vi "test Get Device ID.vi"(11 "Test Case In":refnum<class "Test PCANBasic.lvclass">) -> (0 "error out":errorcluster, 3 "Test Case Out":refnum<class "Test PCANBasic.lvclass">)   [LabVIEW 2020, in "Test PCANBasic.lvclass"]
uses:
  Test PCANBasic.lvclass
  C:/Program Files/National Instruments/LabVIEW 2025/vi.lib/Astemes/LUnit/Test Case.lvclass
  <vilib>/Astemes/LUnit/Test Case.lvclass/Test Case.ctl
  source/PCANBasic.lvlib
  Global PCAN Channel.vi
  <vilib>/Astemes/LUnit/Test Case.lvclass
panel:
  out "Device ID":u32
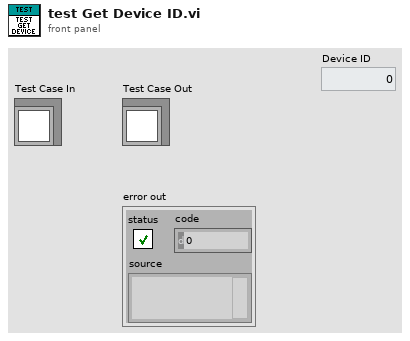
[diagram p1: front panel]
types:
  T1 = typedef "PCANBasic.lvlib/TPCANHandle.ctl" = u16
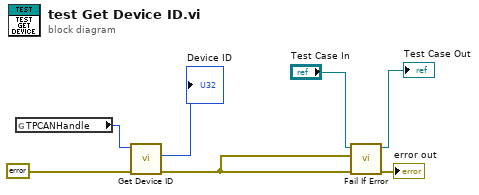
[diagram p0: block diagram]
diagram:
  n1 = global read "Global PCAN Channel.vi" "TPCANHandle"() -> (w2:T1)
  n2 = call "Get Device ID.vi"("error in"=errorcluster {"status"=FALSE, "code"=0, "source"=""}, "TPCANHandle in"=w2) -> ("error out"=w1:errorcluster, "Device ID"=→"Device ID":u32)  [unwired: 6 in, 2 out]
  n3 = call <vilib>:"Fail If Error.vi"("error in (no error)"=w1, "Assert error"=w1, "LUnit Test Case In"="Test Case In") -> ("error out"=→"error out":errorcluster, "LUnit Test Case Out"=→"Test Case Out":refnum<class "Test PCANBasic.lvclass">)  [unwired: 7 in]
